vi "AImain.vi"() -> ()   [LabVIEW 2018]
panel:
  out "substring":string
  out "substring 2":string
  out "Array 10":i32[](array[numeric])
  out "Array 9":i32[](array[numeric])
  out "Array 8":dbl[](array[numeric])
  out "Array 7":dbl[](array[numeric])
  out "Numeric 2":dbl
  out "Falling places":i32
  out "Found":bool
  out "Rotate num":dbl
  out "Numeric":dbl
  out "Array 6":i32[](array[numeric])
  out "subarray 2":i32[](array[numeric])
  out "Array 5":dbl[](array[numeric])
  out "Array 4":i32[][](array[numeric])
  out "size(s)":i32[](array[numeric])
  out "Array 2":dbl[](array[numeric])
  out "error out 16":errorcluster
  out "error out 15":errorcluster
  out "error out 14":errorcluster
  out "error out 13":errorcluster
  out "error out 12":errorcluster
  out "error out 11":errorcluster
  out "error out 10":errorcluster
  out "error out 9":errorcluster
  out "error out 8":errorcluster
  out "error out 7":errorcluster
  out "error out 6":errorcluster
  out "error out 5":errorcluster
  out "error out 4":errorcluster
  out "Boolean":bool
  out "Password":string="tetris"
  out "Array":i32[][](array[numeric])
  out "Next Piece":picture
  out "Score":u32
  out "Rows Cleared":u16
  in  "Difficulty":u16(ring) items=["Easy", "Medium", "Hard"]
  out "Board":picture
  out "error out 2":errorcluster
  out "error out":errorcluster
  in  "?":bool
  out "wait mS":u16=250
  # "AI BASED TETRIS"
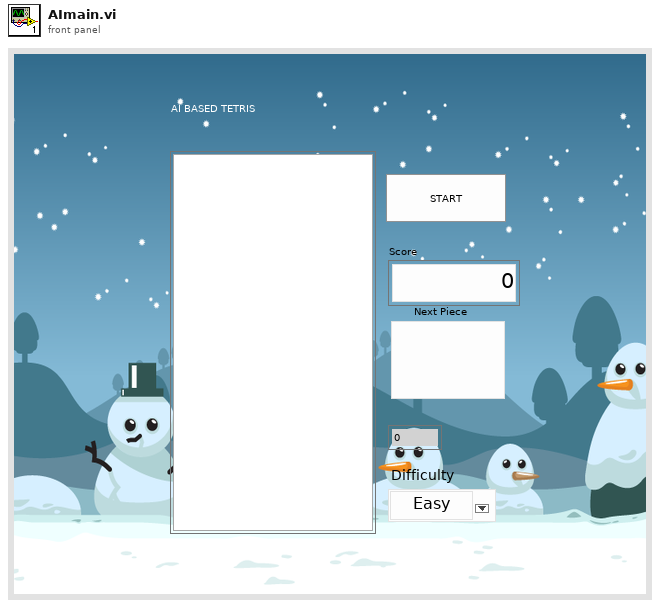
[diagram p1: front panel]
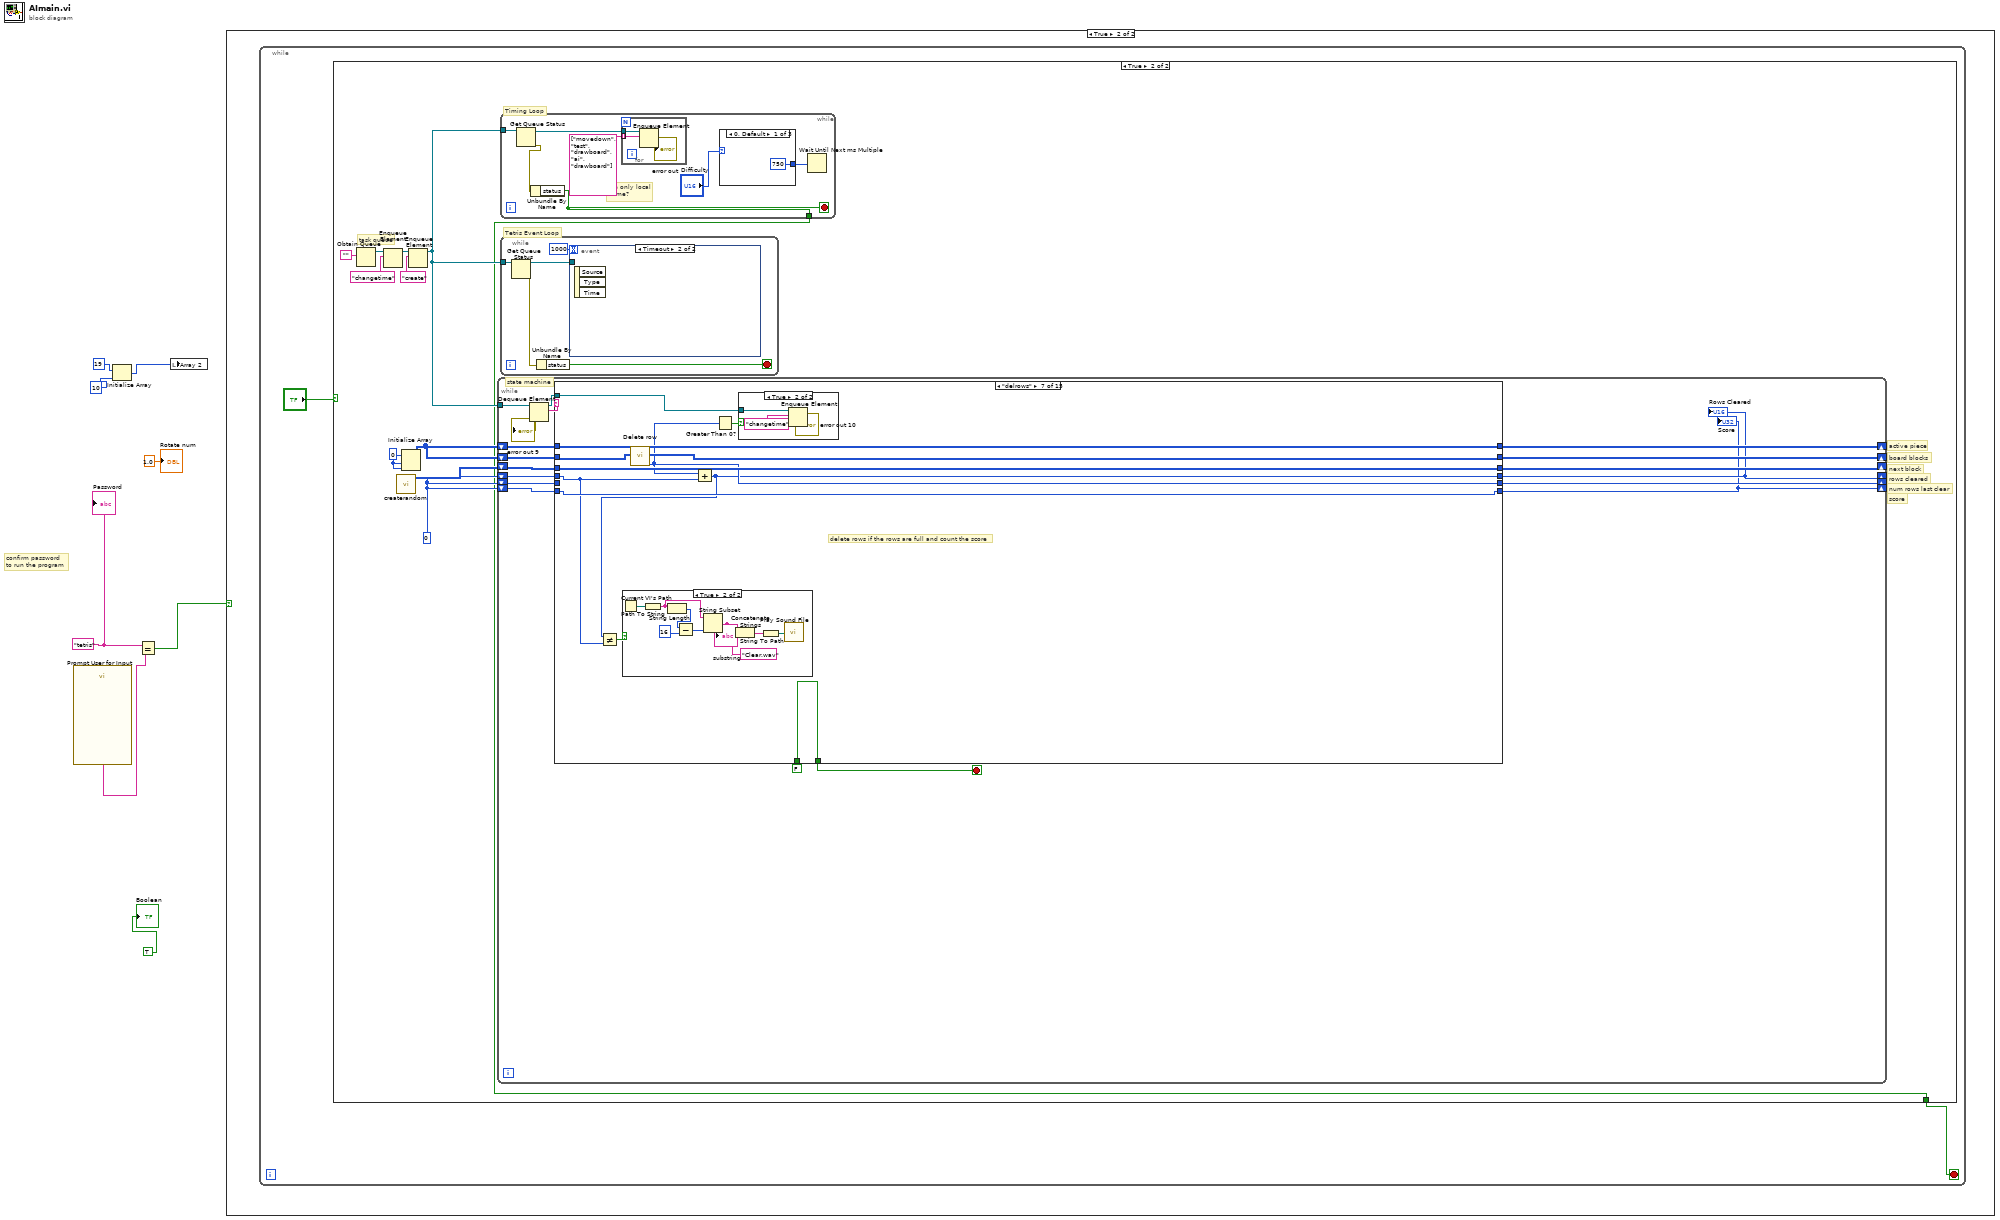
[diagram p0: block diagram]
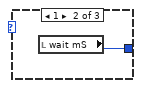
[diagram p4: hidden frame]
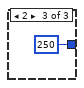
[diagram p5: hidden frame]
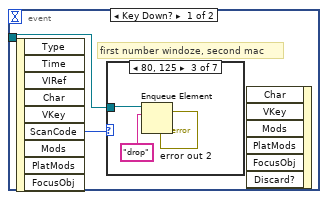
[diagram p6: hidden frame]
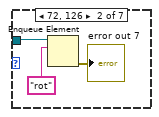
[diagram p8: hidden frame]
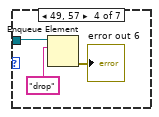
[diagram p9: hidden frame]
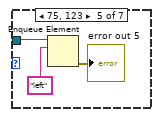
[diagram p10: hidden frame]
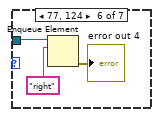
[diagram p11: hidden frame]
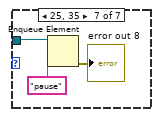
[diagram p12: hidden frame]
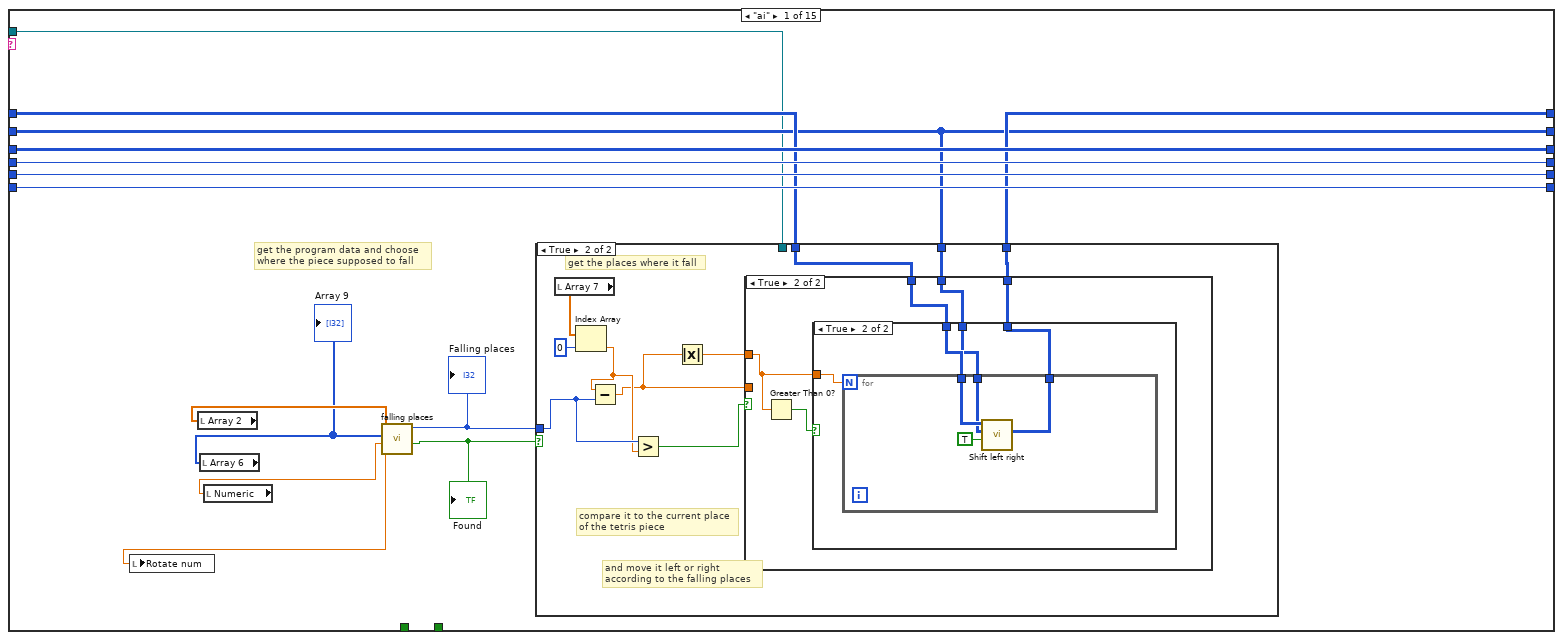
[diagram p13: hidden frame]
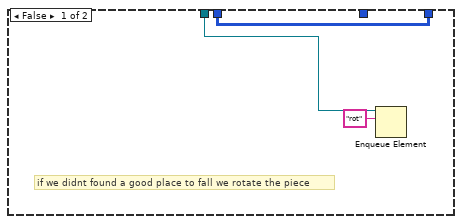
[diagram p14: hidden frame]
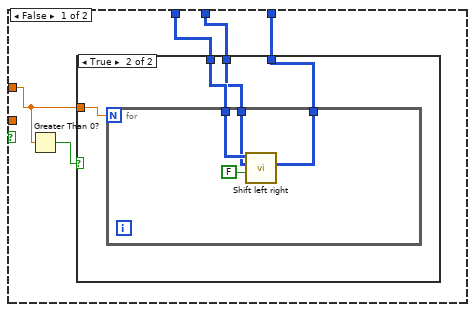
[diagram p15: hidden frame]
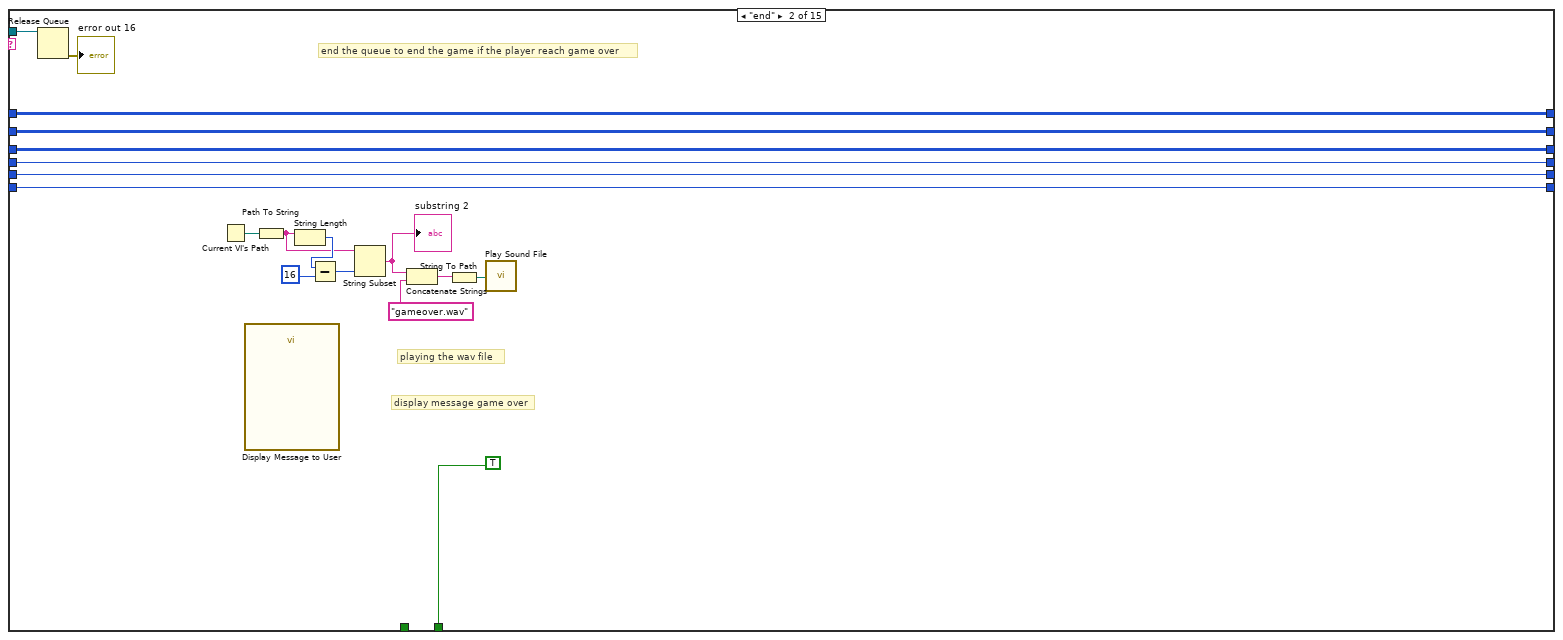
[diagram p18: hidden frame]
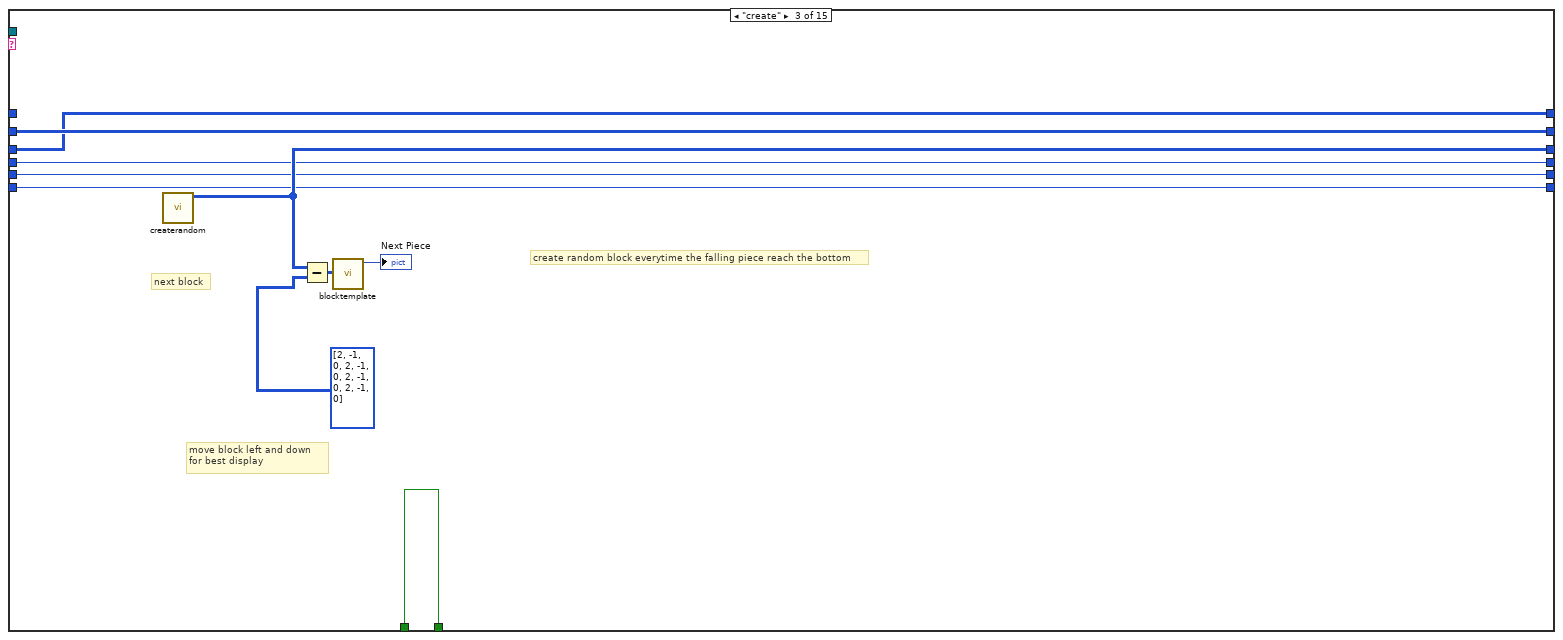
[diagram p19: hidden frame]
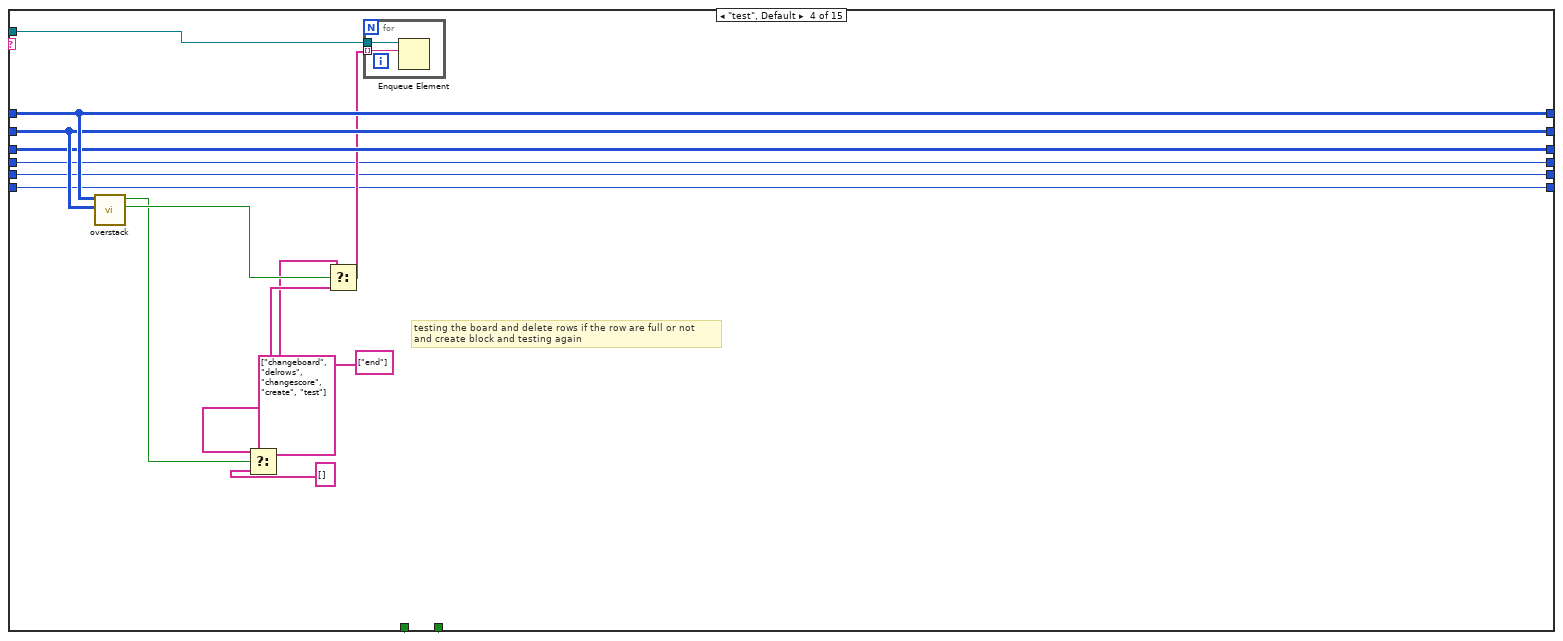
[diagram p20: hidden frame]
diagram:
  w7 = "tetris" ("String")
  # "confirm password \nto run the program"
  n1 = call "Prompt User for Input"() -> ("Input password"=w8:string)  [unwired: 17 in, 2 out]
  n2 = Initialize Array(19, 10) -> (w2:i32[])
  n3 = Equal?(x=w7, y=w8) -> (x = y?=w6:bool)
  n4 = local write "Array 2"(w2) -> ()
  n5 = case shown="True" w6 {
    frame False {
    }
    frame True {
      n6 = while {
        stop <- w9 stop-if-true
        n7 = case shown="True" "?" {
          tunnel: [_ w11] -> w9
          frame False {
          }
          frame True {
            w12 = 0
            w20 = 0
            # "task queue"
            # "num rows last clear"
            # "score"
            # "rows cleared"
            # "Timing Loop"
            # "Tetris Event Loop"
            # "state machine"
            # "next block"
            # "board blocks"
            # "active piece"
            n8 = Obtain Queue(element data type="") -> (queue out=w18:refnum<queue>)  [unwired: 4 in, 2 out]
            n9 = Enqueue Element(queue=w18, element="changetime") -> (queue out=w15:refnum<queue>)  [unwired: 2 in, 2 out]
            n10 = call "createrandom.vi"() -> ("Array"=w21:i32[][])  [unwired: 11 in]
            n11 = Initialize Array(w20, w20, w20) -> (w16:i32[][])
            n12 = Enqueue Element(queue=w15, element="create") -> (queue out=w14:refnum<queue>)  [unwired: 2 in, 2 out]
            n13 = while {
              shift-right: [w67] -> _
              shift-left: w16 -> [w75]
              shift-right: [w68] -> _
              shift-left: w16 -> [w74]
              shift-right: [w72] -> _
              shift-left: w21 -> [w73]
              tunnel: w14 -> [w71]
              shift-right: [w65] -> _
              shift-left: w12 -> [w66]
              shift-right: [w62] -> _
              shift-left: w12 -> [w63]
              shift-right: [w61] -> _
              shift-left: w12 -> [w64]
              stop <- w76 stop-if-true
              n14 = Dequeue Element(queue=w71) -> (queue out=w70:refnum<queue>, element=w69:string, error out=→"error out 9":errorcluster)  [unwired: 2 in, 1 out]
              n15 = case shown="\"delrows\"" w69 {
                tunnel: FALSE -> [_ _ w151 w175 w185 _ w313 w340 w352 w359 w370 w392 w407 w419 w432]
                tunnel: [_ TRUE w151 w175 w185 _ w313 w340 w352 w359 w370 w392 w407 w419 w432] -> w76
                tunnel: [w81 w149 w159 w174 w183 w198 w312 w339 w354 w360 w368 w386 w399 w416 w430] -> w67
                tunnel: w75 -> [w80 w149 _ w174 w183 w198 w312 w339 w354 w362 w368 w387 w401 w417 w430]
                tunnel: w74 -> [w79 w148 w160 w173 w184 w202 w311 w337 w353 w363 w371 w385 w400 w415 w429]
                tunnel: [w79 w148 w160 w173 w182 w202 w310 w337 w353 w363 w371 w385 w400 w415 w429] -> w68
                tunnel: w73 -> [w85 w147 w159 w169 w181 w210 w309 w338 w351 w358 w369 w391 w406 w418 w431]
                tunnel: [w85 w147 w158 w169 w181 w210 w309 w338 w351 w358 w369 w391 w406 w418 w431] -> w72
                tunnel: w70 -> [w78 w143 _ w168 _ _ w308 _ _ _ w367 w382 w397 w408 w426]
                tunnel: [w84 w146 w154 w163 w180 w208 w304 w335 w348 w357 w366 w390 w405 w414 w424] -> w65
                tunnel: w66 -> [w84 w146 w154 w163 w180 w208 w303 w335 w348 w357 w366 w390 w405 w414 w424]
                tunnel: [w83 w145 w153 w162 w179 w207 w305 w334 w346 w356 w365 w389 w404 w413 w423] -> w62
                tunnel: [w82 w144 w152 w161 w178 w206 w307 w336 w342 w355 w364 w388 w403 w412 w422] -> w61
                tunnel: w64 -> [w82 w144 w152 w161 w178 w206 w307 w336 w350 w355 w364 w388 w403 w412 w422]
                tunnel: w63 -> [w83 w145 w153 w162 w179 w207 _ w334 w346 w356 w365 w389 w404 w413 w423]
                frame "ai" {
                  # "get the program data and choose\nwhere the piece supposed to fall"
                  n16 = local read "Array 2"() -> (w91:dbl[])
                  n17 = local read "Array 6"() -> (w90:i32[])
                  "Array 9" <- w90
                  n18 = local read "Numeric"() -> (w89:dbl)
                  n19 = call "falling places.vi"("Size"=w89, "Piece Layer"=w90, "Terrain"=w91) -> ("Found"=w87:bool, "Falling places"=w86:i32, "rotate num"=w88:dbl)  [unwired: 6 in]
                  "Found" <- w87
                  "Falling places" <- w86
                  n20 = local write "Rotate num"(w88) -> ()
                  n21 = case shown="True" w87 {
                    tunnel: w86 -> [_ w99]
                    tunnel: w80 -> [w94 w101]
                    tunnel: [w94 w100] -> w81
                    tunnel: w79 -> [_ w96]
                    tunnel: w78 -> [w93 _]
                    frame False {
                      # "if we didnt found a good place to fall we rotate the piece"
                      n22 = Enqueue Element(queue=w93, element="rot") -> ()  [unwired: 2 in, 3 out]
                    }
                    frame True {
                      # "and move it left or right\naccording to the falling places"
                      # "compare it to the current place\nof the tetris piece"
                      # "get the places where it fall"
                      n23 = local read "Array 7"() -> (w103:dbl[])
                      n24 = Index Array(array=w103, index=0) -> (element=w98:dbl)
                      n25 = Subtract(x=w98, y=w99) -> (x-y=w95:dbl)
                      n26 = Greater?(x=w99, y=w98) -> (0:w97:bool)
                      n27 = Absolute Value(x=w95) -> (abs(x)=w102:dbl)
                      n28 = case shown="True" w97 {
                        tunnel: w102 -> [w106 w119]
                        tunnel: w101 -> [w109 w123]
                        tunnel: [w108 w122] -> w100
                        tunnel: w96 -> [w107 w121]
                        tunnel: w95 -> [_ _]
                        frame False {
                          n29 = Greater Than 0?(x=w106) -> (x > 0?=w105:bool)
                          n30 = case shown="True" w105 {
                            tunnel: w106 -> [_ w114]
                            tunnel: w109 -> [w110 w113]
                            tunnel: [w110 w112] -> w108
                            tunnel: w107 -> [_ w111]
                            frame False {
                            }
                            frame True {
                              n31 = for {
                                N: w114 -> [_]
                                tunnel: w113 -> [w118]
                                tunnel: [w117] -> w112
                                tunnel: w111 -> [w115]
                                n32 = call "Shift left right.vi"("TETRIS BLOCK"=w118, "Filled Array"=w115, "Move Right"=FALSE) -> ("After Shift"=w117:u8[][])  [unwired: 6 in]
                              }
                            }
                          }
                        }
                        frame True {
                          n33 = Greater Than 0?(x=w119) -> (x > 0?=w120:bool)
                          n34 = case shown="True" w120 {
                            tunnel: w119 -> [_ w128]
                            tunnel: w123 -> [w124 w127]
                            tunnel: [w124 w126] -> w122
                            tunnel: w121 -> [_ w125]
                            frame False {
                            }
                            frame True {
                              n35 = for {
                                N: w128 -> [_]
                                tunnel: w127 -> [w132]
                                tunnel: [w131] -> w126
                                tunnel: w125 -> [w129]
                                n36 = call "Shift left right.vi"("TETRIS BLOCK"=w132, "Filled Array"=w129, "Move Right"=TRUE) -> ("After Shift"=w131:u8[][])  [unwired: 6 in]
                              }
                            }
                          }
                        }
                      }
                    }
                  }
                }
                frame "end" {
                  # "display message game over"
                  # "playing the wav file"
                  # "end the queue to end the game if the player reach game over"
                  n37 = Release Queue(queue=w143) -> (error out=→"error out 16":errorcluster)  [unwired: 2 in, 2 out]
                  n38 = Current VI's Path() -> (path=w140:path)
                  n39 = call "Display Message to User"() -> ()  [unwired: 10 in, 2 out]
                  n40 = Path To String(path=w140) -> (string=w133:string)
                  n41 = String Length(string=w133) -> (length=w137:i32)
                  n42 = Subtract(x=w137, y=16) -> (x-y=w135:i32)
                  n43 = String Subset(string=w133, length (rest)=w135) -> (substring=w134:string)  [unwired: 1 in]
                  "substring 2" <- w134
                  n44 = Concatenate Strings(w134, "gameover.wav" ("string")) -> (w141:string)
                  n45 = String To Path(string=w141) -> (path=w139:path)
                  n46 = call <vilib>:"Play Sound File.vi"("path"=w139) -> ()  [unwired: 9 in, 2 out]
                }
                frame "create" {
                  # "create random block everytime the falling piece reach the bottom"
                  # "move block left and down\nfor best display"
                  # "next block"
                  n47 = call "createrandom.vi"() -> ("Array"=w158:i32[][])  [unwired: 11 in]
                  n48 = Subtract(x=w158, y=i32[][] [[2, -1, 0], [2, -1, 0], [2, -1, 0], [2, -1, 0]]) -> (x-y=w156:i32[][])
                  n49 = call "blocktemplate.vi"("Piece Array"=w156) -> ("Picture"=→"Next Piece":picture)  [unwired: 10 in]
                }
                frame "test", Default {
                  # "testing the board and delete rows if the row are full or not \nand create block and testing again"
                  n50 = call "overstack.vi"("board array"=w173, "Piece Array"=w174) -> ("Lost"=w171:bool, "Touching"=w170:bool)  [unwired: 7 in, 1 out]
                  n51 = Select(t=string[] ["changeboard", "delrows", "changescore", "create", "test"], s=w170, f=string[] []) -> (s? t:f=w172:string[])
                  n52 = Select(t=string[] ["end"], s=w171, f=w172) -> (s? t:f=w167:string[])
                  n53 = for {
                    tunnel: w168 -> [w177]
                    tunnel: w167 -> [w176] mode=indexing
                    n54 = Enqueue Element(queue=w177, element=w176) -> ()  [unwired: 2 in, 3 out]
                  }
                }
                frame "changeboard" {
                  # "change board case"
                  n55 = Build Array (concatenate)(w184, w183) -> (w182:i32[][])
                }
                frame "drawboard" {
                  w194 = 0.0
                  # "get the data of the current falling piece on the time\nthe program drawing tetris board\nand pass it to get data for the AI to work with"
                  # "drawboard and get the data of the falling piece"
                  n56 = Initialize Array(-1.0 ("element"), 4 ("dimension size")) -> (→"Array 5":dbl[])
                  n57 = call "blocktemplate.vi"("Piece Array"=w198, "board array"=w202) -> ("Picture"=→"Board":picture)  [unwired: 9 in]
                  n58 = for {
                    N: 4 -> [_]
                    tunnel: [w261] -> w193
                    i -> [w262]
                    n59 = for {
                      N: 4 -> [_]
                      tunnel: w262 -> [w289]
                      tunnel: [w286] -> w268 mode=indexing
                      tunnel: [w285] -> w264
                      tunnel: [w284] -> w265
                      i -> [w288]
                      n60 = local read "Array 5"() -> (w287:dbl[])
                      n61 = local read "subarray 2"() -> (w290:i32[])
                      n62 = Index Array(array=w287, index=w288) -> (element=w284:dbl)
                      n63 = Index Array(array=w290, index=w289) -> (element=w285:i32)
                      n64 = Not Equal?(x=w285, y=w284) -> (x != y?=w286:bool)
                    }
                    n65 = Equal?(x=w262, y=3.0) -> (x = y?=w261:bool)
                    n66 = And Array Elements(Boolean array=w268) -> (logical AND=w266:bool)
                    n67 = Select(t=w264, s=w266, f=w265) -> (s? t:f=w267:dbl)
                    n68 = case shown="True" w266 {
                      tunnel: w267 -> [_ w270]
                      frame False {
                      }
                      frame True {
                        n69 = local read "Array 5"() -> (w271:dbl[])
                        n70 = while {
                          tunnel: w271 -> [w277] mode=indexing
                          tunnel: w271 -> [w275]
                          tunnel: w270 -> [w274]
                          i -> [w273]
                          stop <- w272 stop-if-true
                          n71 = Equal?(x=w277, y=-1.0) -> (x = y?=w276:bool)
                          n72 = case shown="True" w276 {
                            tunnel: w275 -> [w283 _]
                            tunnel: w274 -> [w282 _]
                            tunnel: w273 -> [w281 _]
                            tunnel: [TRUE _] -> w272
                            frame True {
                              n73 = Replace Array Subset(array=w283, new element=w282, index=w281) -> (w280:dbl[])
                              n74 = local write "Array 5"(w280) -> ()
                            }
                            frame False {
                            }
                          }
                        }
                      }
                    }
                  }
                  n75 = Index Array(array=w198, index (col)=0 ("disabled index (col)")) -> (element=→"subarray 2":i32[])  [unwired: 1 in]
                  n76 = Array Size(array=w202) -> (size(s)=w205:i32[])
                  "size(s)" <- w205
                  n77 = Index Array(array=w205, index=0) -> (element=w203:i32)
                  n78 = for {
                    N: w203 -> [_]
                    tunnel: w202 -> [w298]
                    i -> [w300]
                    n79 = Index Array(array=w298, index (row)=w300, index (col)=0 ("disabled index (col)")) -> (element=w295:i32)
                    n80 = local read "Array 2"() -> (w296:dbl[])
                    n81 = Index Array(array=w296, index=w295) -> (element=w291:dbl)
                    n82 = Index Array(array=w298, index (row)=w300, index (col)=1) -> (element=w292:i32)
                    n83 = Greater?(x=w291, y=w292) -> (0:w297:bool)
                    n84 = Select(t=w292, s=w297, f=w291) -> (s? t:f=w293:dbl)
                    n85 = Replace Array Subset(array=w296, new element=w293, index=w295) -> (→"Array 2":dbl[])
                  }
                  n86 = case shown="True" w193 {
                    tunnel: [_ w215] -> w192
                    frame False {
                    }
                    frame True {
                      n87 = for {
                        N: 4 -> [_]
                        tunnel: [w219] -> w217
                        i -> [w219]
                        n88 = local read "Array 5"() -> (w223:dbl[])
                        n89 = Index Array(array=w223, index=w219) -> (element=w222:dbl)
                        n90 = Equal?(x=w222, y=-1.0) -> (x = y?=w220:bool)
                        n91 = case shown="False" w220 {
                          frame False {
                            n92 = local read "Numeric 2"() -> (w226:dbl)
                            n93 = Add(x=w226, y=1.0) -> (x+y=w224:dbl)
                            n94 = local write "Numeric 2"(w224) -> ()
                          }
                          frame True {
                          }
                        }
                      }
                      n95 = Equal?(x=w217, y=3) -> (x = y?=w215:bool)
                    }
                  }
                  n96 = case shown="True" w192 {
                    tunnel: [_ TRUE] -> w191
                    tunnel: [_ w212] -> w190
                    tunnel: [_ w211] -> w188
                    frame False {
                    }
                    frame True {
                      n97 = local read "Numeric 2"() -> (w211:dbl)
                      n98 = local read "Array 5"() -> (w212:dbl[])
                      n99 = Array Subset(array=w212, index=1, length=w211) -> ()  [unwired: 1 out]
                    }
                  }
                  "Array 8" <- w190
                  n100 = Array Subset(array=w190, index=0, length=w188) -> (w187:dbl[])
                  "Array 7" <- w187
                  n101 = Sort 1D Array(array=w187) -> (sorted array=w186:dbl[])
                  n102 = local write "Array 7"(w186) -> ()
                  n103 = case shown="True" w191 {
                    frame False {
                    }
                    frame True {
                      n104 = local read "Array 7"() -> (w227:dbl[])
                      n105 = for {
                        N: 4 -> [_]
                        tunnel: w227 -> [w247]
                        tunnel: [w244] -> w229 mode=indexing
                        tunnel: [w241] -> w228
                        i -> [w243]
                        n106 = for {
                          N: 4 -> [_]
                          tunnel: w247 -> [w256]
                          tunnel: w243 -> [w255]
                          tunnel: [w248] -> w245 mode=indexing
                          i -> [w249]
                          n107 = local read "Array 4"() -> (w250:i32[][])
                          n108 = Index Array(array=w256, index=w255) -> (element=w253:dbl)
                          n109 = Index Array(array=w250, index (row)=w249, index (col)=0 ("disabled index (col)")) -> (element=w252:i32)
                          n110 = Equal?(x=w253, y=w252) -> (x = y?=w251:bool)
                          n111 = case shown="True" w251 {
                            tunnel: w250 -> [_ w260]
                            tunnel: w249 -> [_ w258]
                            tunnel: [_ w257] -> w248
                            frame False {
                            }
                            frame True {
                              n112 = Index Array(array=w260, index (row)=w258, index (col)=1 ("disabled index (col)")) -> (element=w257:i32)
                            }
                          }
                        }
                        "Array 10" <- w245
                        n113 = Equal?(x=w243, y=3) -> (x = y?=w241:bool)
                        n114 = Array Max & Min(array=w245) -> (max value=w244:i32)  [unwired: 3 out]
                      }
                      "Array 6" <- w229
                      n115 = case shown="True" w228 {
                        frame False {
                        }
                        frame True {
                          n116 = local read "Array 6"() -> (w231:i32[])
                          n117 = for {
                            N: 4 -> [_]
                            tunnel: w231 -> [w236]
                            i -> [w237]
                            n118 = Index Array(array=w236, index=w237) -> (element=w234:i32)
                            n119 = Not Equal?(x=w234, y=0.0) -> (x != y?=w233:bool)
                            n120 = case shown="True" w233 {
                              frame False {
                              }
                              frame True {
                                n121 = local read "Numeric"() -> (w240:dbl)
                                n122 = Add(x=w240, y=1.0) -> (x+y=w238:dbl)
                                n123 = local write "Numeric"(w238) -> ()
                              }
                            }
                          }
                        }
                      }
                    }
                  }
                  "Array" <- w202
                  "Array 4" <- w198
                  "Numeric" <- w194
                  "Numeric 2" <- w194
                }
                frame "delrows" {
                  # "delete rows if the rows are full and count the score"
                  n124 = call "Delete row.vi"("tetris block"=w311) -> ("Rows Deleted"=w305:u16, "new tetris block"=w310:u8[][])  [unwired: 9 in]
                  n125 = Add(x=w305, y=w303) -> (x+y=w304:i32)
                  n126 = Not Equal?(x=w304, y=w303) -> (x != y?=w302:bool)
                  n127 = case shown="True" w302 {
                    frame False {
                    }
                    frame True {
                      n128 = Current VI's Path() -> (path=w321:path)
                      n129 = Path To String(path=w321) -> (string=w315:string)
                      n130 = String Length(string=w315) -> (length=w318:i32)
                      n131 = Subtract(x=w318, y=16) -> (x-y=w316:i32)
                      n132 = String Subset(string=w315, length (rest)=w316) -> (substring=w314:string)  [unwired: 1 in]
                      "substring" <- w314
                      n133 = Concatenate Strings(w314, "Clear.wav" ("string")) -> (w322:string)
                      n134 = String To Path(string=w322) -> (path=w320:path)
                      n135 = call <vilib>:"Play Sound File.vi"("path"=w320) -> ()  [unwired: 9 in, 2 out]
                    }
                  }
                  n136 = Greater Than 0?(x=w305) -> (x > 0?=w306:bool)
                  n137 = case shown="True" w306 {
                    tunnel: w308 -> [_ w324]
                    frame False {
                    }
                    frame True {
                      n138 = Enqueue Element(queue=w324, element="changetime") -> (error out=→"error out 10":errorcluster)  [unwired: 2 in, 2 out]
                    }
                  }
                }
                frame "changetime" {
                  w329 = 100
                  w332 = 10
                  # "start time"
                  # "wait time the only local in this example"
                  n139 = Quotient & Remainder(x=w335, y=w332) -> (floor(x/y)=w333:i32)  [unwired: 1 out]
                  n140 = Multiply(x=w333, y=w332) -> (x*y=w331:i32)
                  n141 = Subtract(x=w329, y=w331) -> (x-y=w330:i32)
                  n142 = Divide(x=w330, y=w329) -> (x/y=w328:dbl)
                  n143 = Multiply(x=w328, y=500) -> (x*y=→"wait mS":dbl)
                }
                frame "changescore" {
                  # "getting the score according to how much the lines cleared at once\nthe more lines clear at once the higher score we get at once"
                  n144 = Index Array(array=i32[] [1, 40, 100, 300, 1200], index=w346) -> (element=w343:i32)
                  n145 = Quotient & Remainder(x=w348, y=10) -> (floor(x/y)=w347:i32)  [unwired: 1 out]
                  n146 = Increment(x=w347) -> (x+1=w344:i32)
                  n147 = Multiply(x=w344, y=w343) -> (x*y=w341:i32)
                  n148 = Add(x=w350, y=w341) -> (x+y=w342:i32)
                }
                frame "movedown" {
                  # "move down one block at a time for\nthe falling piece"
                  n149 = Add(x=w362, y=i32[][] [[0, 1, 0], [0, 1, 0], [0, 1, 0], [0, 1, 0]]) -> (x+y=w360:i32[][])
                }
                frame "pause" {
                  # "to pause thte game"
                  # "pop values off the stack\nchecking for \"pause\""
                  n150 = while {
                    tunnel: w367 -> [w377]
                    stop <- w374 stop-if-true
                    n151 = Dequeue Element(queue=w377) -> (element=w375:string, error out=→"error out 11":errorcluster)  [unwired: 2 in, 2 out]
                    n152 = Wait (ms)(milliseconds to wait=25) -> ()  [unwired: 1 out]
                    n153 = Equal?(x=w375, y="pause") -> (x = y?=w374:bool)
                  }
                }
                frame "right" {
                  # "move the faliing piece to the right"
                  n154 = Enqueue Element(queue=w382, element="test") -> (queue out=w380:refnum<queue>, error out=→"error out 15":errorcluster)  [unwired: 2 in, 1 out]
                  n155 = Enqueue Element(queue=w380, element="drawboard") -> (error out=→"error out 14":errorcluster)  [unwired: 2 in, 2 out]
                  n156 = call "Shift left right.vi"("TETRIS BLOCK"=w387, "Filled Array"=w385, "Move Right"=TRUE) -> ("After Shift"=w386:u8[][])  [unwired: 6 in]
                }
                frame "left" {
                  # "move the falling piece to the left using the same vi but \ndifferent input"
                  n157 = Enqueue Element(queue=w397, element="test") -> (queue out=w396:refnum<queue>, error out=→"error out 12":errorcluster)  [unwired: 2 in, 1 out]
                  n158 = Enqueue Element(queue=w396, element="drawboard") -> (error out=→"error out 13":errorcluster)  [unwired: 2 in, 2 out]
                  n159 = call "Shift left right.vi"("TETRIS BLOCK"=w401, "Filled Array"=w400, "Move Right"=FALSE) -> ("After Shift"=w399:u8[][])  [unwired: 6 in]
                }
                frame "rot" {
                  # "rotate the piece and drawboard again once it rotated to get the visual data"
                  n160 = Enqueue Element(queue=w408, element="test") -> (queue out=w410:refnum<queue>)  [unwired: 2 in, 2 out]
                  n161 = Enqueue Element(queue=w410, element="drawboard") -> ()  [unwired: 2 in, 3 out]
                  n162 = call "rotate.vi"(9:w415, 11:w417) -> (3:w416:u8[][])  [unwired: 9 in]
                }
                frame "drop" {
                  # "drop the piece by first counting the range of the falling piece\nto the stack and move it down according to the range."
                  n163 = call "overstack.vi"("board array"=w429, "Piece Array"=w430) -> ("min Distance"=w421:i16)  [unwired: 7 in, 2 out]
                  n164 = Decrement(x=w421) -> (x-1=w420:i16)
                  n165 = for {
                    N: w420 -> [_]
                    tunnel: ["movedown"] -> w428 mode=indexing
                  }
                  n166 = Build Array (concatenate)(w428, "test") -> (w425:string[])
                  n167 = for {
                    tunnel: w426 -> [w434]
                    tunnel: w425 -> [w433] mode=indexing
                    n168 = Enqueue Element(queue=w434, element=w433) -> ()  [unwired: 2 in, 3 out]
                  }
                }
              }
              "Rows Cleared" <- w65
              "Score" <- w61
            }
            n169 = while {
              tunnel: w14 -> [w26]
              tunnel: [w22] -> w11
              stop <- w22 stop-if-true
              # "the only local\nfixme?"
              n170 = Get Queue Status(queue=w26) -> (queue out=w25:refnum<queue>, error out=w27:errorcluster)  [unwired: 2 in, 6 out]
              n171 = Unbundle By Name(w27) -> ("status"=w22:bool)
              n172 = for {
                tunnel: w25 -> [w34]
                tunnel: string[] ["movedown", "test", "drawboard", "ai", "drawboard"] -> [w33] mode=indexing
                n173 = Enqueue Element(queue=w34, element=w33) -> (error out=→"error out":errorcluster)  [unwired: 2 in, 2 out]
              }
              n174 = case shown="0, Default" "Difficulty" {
                tunnel: [u16 750 ("wait mS") w30 u16 250 ("wait mS")] -> w24
                frame 0, Default {
                }
                frame 1 {
                  n175 = local read "wait mS"() -> (w30:u16)
                }
                frame 2 {
                }
              }
              n176 = Wait Until Next ms Multiple(millisecond multiple=w24) -> ()  [unwired: 1 out]
            }
            n177 = while {
              tunnel: w14 -> [w36]
              stop <- w37 stop-if-true
              n178 = Get Queue Status(queue=w36) -> (queue out=w35:refnum<queue>, error out=w38:errorcluster)  [unwired: 2 in, 6 out]
              n179 = Unbundle By Name(w38) -> ("status"=w37:bool)
              n180 = event shown="[1] Timeout" {
                selector: _ -> [_ _]
                dyn-events: _ -> [_ _]
                timeout: 1000 -> [_ _]
                tunnel: w35 -> [w40 _]
                event Key Down? {
                  # "first number windoze, second mac"
                  n181 = event-data() -> ("ScanCode"=w41:i16)  [unwired: 1 in, 8 out]
                  n182 = case shown="80, 125" w41 {
                    tunnel: w40 -> [_ w44 w47 w50 w53 w56 w59]
                    frame 0, Default {
                    }
                    frame 72, 126 {
                      n183 = Enqueue Element(queue=w44, element="rot") -> (error out=→"error out 7":errorcluster)  [unwired: 2 in, 2 out]
                    }
                    frame 80, 125 {
                      n184 = Enqueue Element(queue=w47, element="drop") -> (error out=→"error out 2":errorcluster)  [unwired: 2 in, 2 out]
                    }
                    frame 49, 57 {
                      n185 = Enqueue Element(queue=w50, element="drop") -> (error out=→"error out 6":errorcluster)  [unwired: 2 in, 2 out]
                    }
                    frame 75, 123 {
                      n186 = Enqueue Element(queue=w53, element="left") -> (error out=→"error out 5":errorcluster)  [unwired: 2 in, 2 out]
                    }
                    frame 77, 124 {
                      n187 = Enqueue Element(queue=w56, element="right") -> (error out=→"error out 4":errorcluster)  [unwired: 2 in, 2 out]
                    }
                    frame 25, 35 {
                      n188 = Enqueue Element(queue=w59, element="pause") -> (error out=→"error out 8":errorcluster)  [unwired: 2 in, 2 out]
                    }
                  }
                  n189 = event-data() -> ()  [unwired: 7 in, 1 out]
                }
                event Timeout {
                  n190 = event-data() -> ()  [unwired: 1 in, 3 out]
                }
              }
            }
          }
        }
      }
    }
  }
  "Password" <- w7
  "Boolean" <- TRUE
  "Rotate num" <- 1.0 ("Numeric 2")
